vi "worksheet set background.vi"(8 "error in (no error)":errorcluster, 10 "filename":string, 11 "worksheet":u32) -> (0 "error out":errorcluster, 3 "function return":u32(ring))   [LabVIEW 8.6]
doc: "lxw_error worksheet_set_background(lxw_worksheet worksheet, const char *filename);"
uses:
  pending_lvxlsxwriter/xlsxwriter.dll
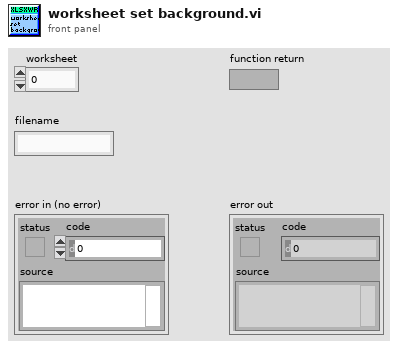
[diagram p1: front panel]
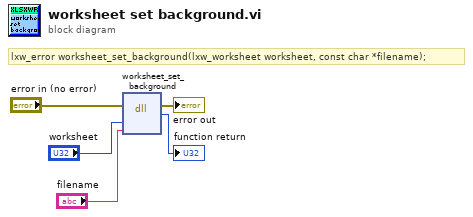
[diagram p0: block diagram]
diagram:
  # "lxw_error worksheet_set_background(lxw_worksheet worksheet, const char *filename);"
  n1 = dll-call lib="C:/Users/WDAGUtilityAccount/Desktop/pending_lvxlsxwriter/xlsxwriter.*" fn="worksheet_set_background"(error in="error in (no error)", "worksheet"="worksheet", "filename"="filename") -> (error out=→"error out":errorcluster, →"function return":u32)  [unwired: 4 in, 1 out]
